vi "TDMS_Saver.vi"(10 "TDMS Cluster":T1, 11 "Data to Log":dbl[](array[numeric])) -> ()   [LabVIEW 2016]
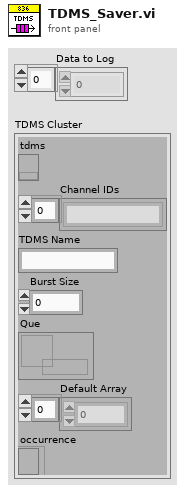
[diagram p1: front panel]
types:
  T1 = cluster{"tdms":refnum<k34>, "Channel IDs":string[], "TDMS Name":string, "Burst Size":i32, "Que":refnum<k33>, "Default Array":dbl[], "occurrence":refnum<k4>}
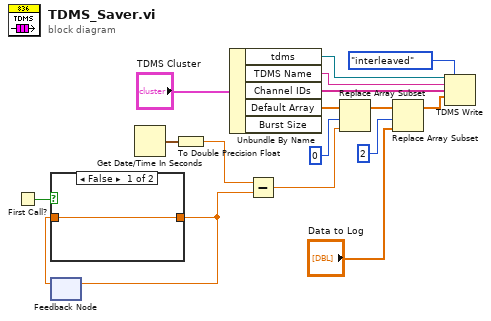
[diagram p0: block diagram]
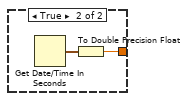
[diagram p2: hidden frame]
diagram:
  n1 = First Call?() -> (First Call?: T/F=w13:bool)
  n2 = feedback #1() -> (w14:dbl)  [unwired: 1 in]
  n3 = case shown="False" w13 {
    tunnel: [w18 w19] -> w15
    tunnel: w14 -> [w18 _]
    frame False {
    }
    frame True {
      n4 = Get Date/Time In Seconds() -> (seconds since 1Jan1904=w20:timestamp)
      n5 = To Double Precision Float(number=w20) -> (double precision float=w19:dbl)
    }
  }
  n6 = feedback-in #1(w15) -> ()
  n7 = Get Date/Time In Seconds() -> (seconds since 1Jan1904=w7:timestamp)
  n8 = To Double Precision Float(number=w7) -> (double precision float=w8:dbl)
  n9 = Unbundle By Name("TDMS Cluster") -> ("tdms"=w3:refnum<k34>, "TDMS Name"=w2:string, "Channel IDs"=w1:string[], "Default Array"=w17:dbl[])  [unwired: 1 out]
  n10 = Subtract(x=w8, y=w15) -> (x-y=w9:dbl)
  n11 = Replace Array Subset(array=w17, new element=w9, index=0) -> (w10:dbl[])
  n12 = Replace Array Subset(array=w10, new element="Data to Log", index=2) -> (w4:dbl[])
  n13 = TDMS Write(0:w3, 1:enum16{"decimated", "interleaved"}."interleaved" ("data layout (0:decimated)"), 5:w2, 7:w1, 9:w4) -> ()  [unwired: 1 in, 4 out]
